vi "Search_Dust_Types.vi"() -> ()   [LabVIEW 2013]
uses:
  Private/Controls/Dust_list.ctl
  <vilib>/Utility/miscctls.llb/LVPointTypeDef.ctl
panel:
  out "Descending":string
  out "Ascending":string
  out "dust_weight text":string
  out "bottle_weight text":string
  out "source_weight text":string
  out "dust_density text":string
  out "dust_name text":string
  out "id_dust_type text":string
  in  "Exit":bool
  out "error out":errorcluster
  in  "error in (no error)":errorcluster
  in  "dust_weight":bool
  in  "bottle_weight":bool
  in  "source_weight":bool
  in  "dust_density":bool
  in  "dust_name":bool
  in  "id_dust_type":bool
  out "Array":T1[](array[typedef])
  # "Size"
  # "Comments"
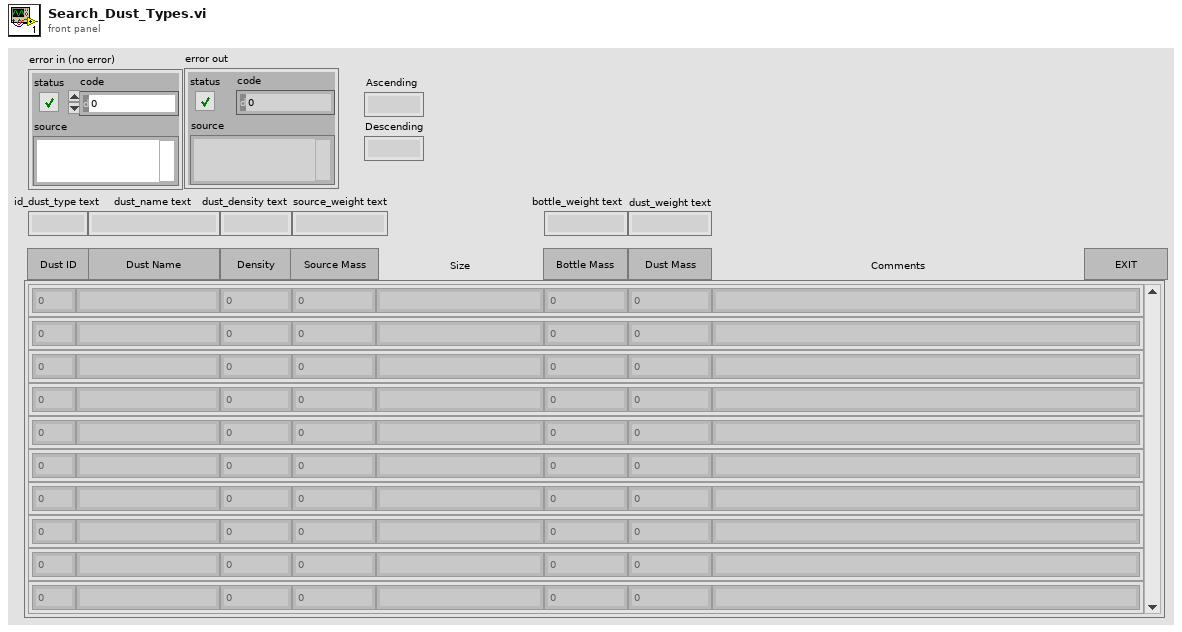
[diagram p1: front panel]
types:
  T1 = typedef "dust_list.ctl" = cluster{"id_dust_type":i32, "dust_name":string, "dust_density":dbl, "source_weight":dbl, "size":string, "bottle_weight":dbl, "dust_mass":dbl, "comments":string}
  T2 = typedef "LVPointTypeDef.ctl" = cluster{"Horizontal":i16, "Vertical":i16}
  T3 = enum16{"dust_name", "dust_density", "source_weight", "bottle_weight", "dust_weight"}
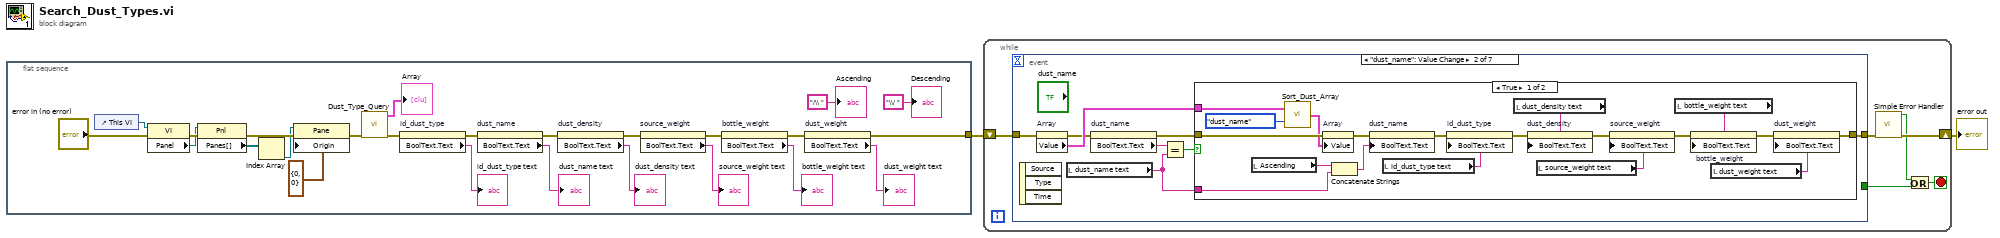
[diagram p0: block diagram]
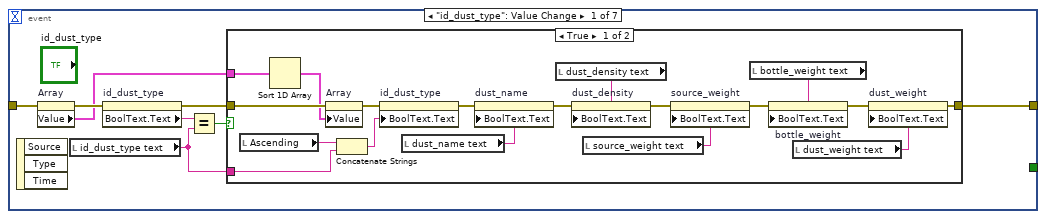
[diagram p2: hidden frame]
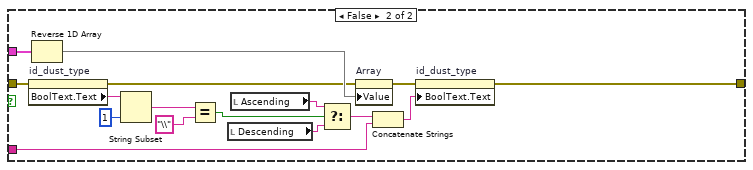
[diagram p3: hidden frame]
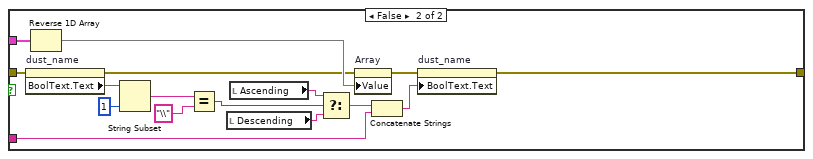
[diagram p4: hidden frame]
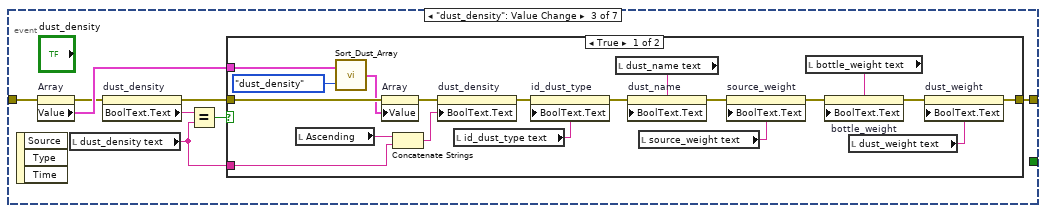
[diagram p5: hidden frame]
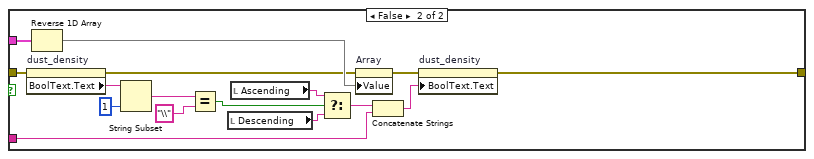
[diagram p6: hidden frame]
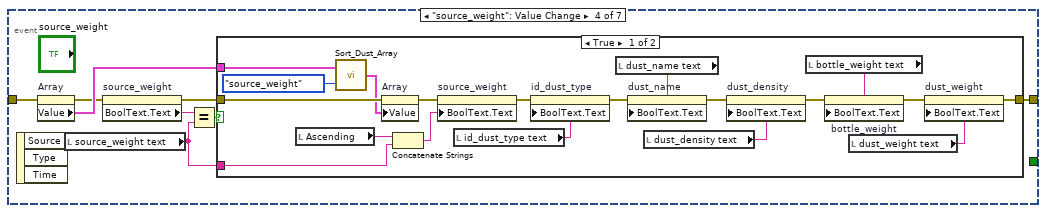
[diagram p7: hidden frame]
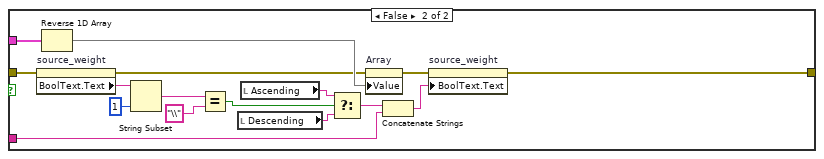
[diagram p8: hidden frame]
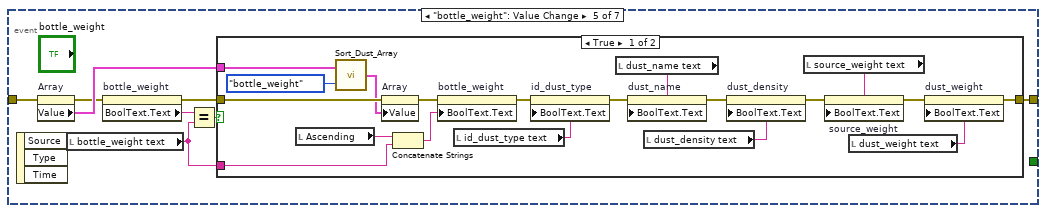
[diagram p9: hidden frame]
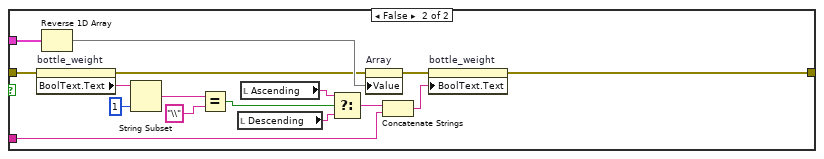
[diagram p10: hidden frame]
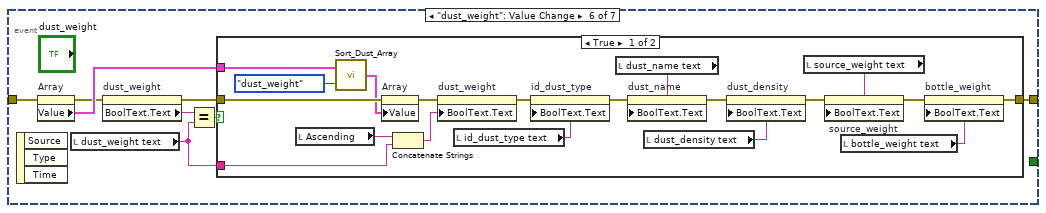
[diagram p11: hidden frame]
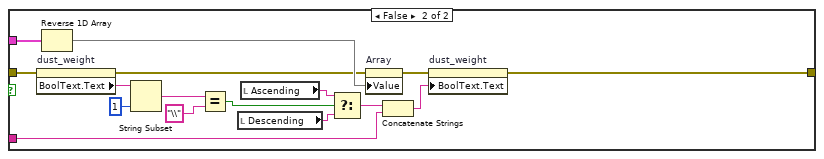
[diagram p12: hidden frame]
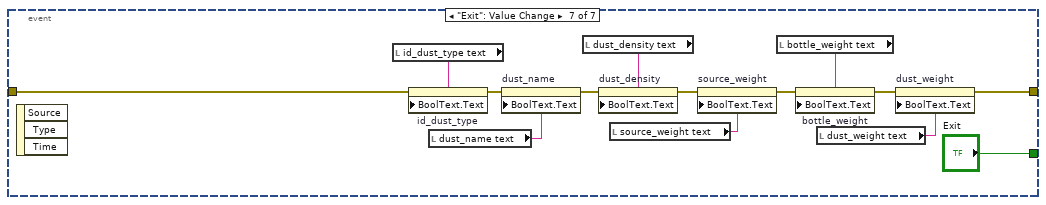
[diagram p13: hidden frame]
diagram:
  n1 = flat-sequence {
    tunnel: [w16] -> w1
    frame #0 {
      n2 = control-ref of="This VI"() -> (w10:refnum<vi>)
      n3 = property class="VI"(reference=w10, error in="error in (no error)") -> (error out=w9:errorcluster, "Panel"=w8:refnum<vi>)  [unwired: 1 out]
      n4 = property class="Pnl"(reference=w8, error in=w9) -> (error out=w7:errorcluster, "Panes[]"=w6:refnum<vi>[])  [unwired: 1 out]
      n5 = Index Array(array=w6) -> (element=w5:refnum<vi>)  [unwired: 1 in]
      n6 = property class="Pane"(reference=w5, error in=w7, "Origin"=T2 {"Horizontal"=0, "Vertical"=0}) -> (error out=w3:errorcluster)  [unwired: 1 out]
      n7 = call "Dust_Type_Query.vi"("error in (no error)"=w3) -> ("error out"=w13:errorcluster, "Dust Type Array"=→"Array":T1[])  [unwired: 9 in]
      n8 = property on="id_dust_type" class="Bool"(error in=w13) -> (error out=w26:errorcluster, "BoolText.Text"=→"id_dust_type text":string)  [unwired: 1 in, 1 out]
      n9 = property on="dust_name" class="Bool"(error in=w26) -> (error out=w25:errorcluster, "BoolText.Text"=→"dust_name text":string)  [unwired: 1 in, 1 out]
      n10 = property on="dust_density" class="Bool"(error in=w25) -> (error out=w22:errorcluster, "BoolText.Text"=→"dust_density text":string)  [unwired: 1 in, 1 out]
      n11 = property on="source_weight" class="Bool"(error in=w22) -> (error out=w20:errorcluster, "BoolText.Text"=→"source_weight text":string)  [unwired: 1 in, 1 out]
      n12 = property on="bottle_weight" class="Bool"(error in=w20) -> (error out=w18:errorcluster, "BoolText.Text"=→"bottle_weight text":string)  [unwired: 1 in, 1 out]
      n13 = property on="dust_weight" class="Bool"(error in=w18) -> (error out=w16:errorcluster, "BoolText.Text"=→"dust_weight text":string)  [unwired: 1 in, 1 out]
      "Ascending" <- "/\\ " ("Ascending")
      "Descending" <- "\\/ " ("Descending")
    }
  }
  n14 = while {
    shift-right: [w30] -> w2
    shift-left: w1 -> [w33]
    stop <- w29 stop-if-true
    n15 = event shown="[1] \"dust_name\": Value Change" {
      selector: _ -> [_ _ _ _ _ _ _]
      dyn-events: _ -> [_ _ _ _ _ _ _]
      timeout: _ -> [_ _ _ _ _ _ _]
      tunnel: w33 -> [w41 w83 w126 w169 w212 w255 w298]
      tunnel: [w40 w82 w125 w168 w211 w254 w297] -> w32
      tunnel: [_ _ _ _ _ _ "Exit"] -> w31
      event "id_dust_type": Value Change {
        n16 = event-data() -> ()  [unwired: 1 in, 3 out]
        n17 = property on="Array" class="Arr (strict)"(error in=w41) -> (error out=w35:errorcluster, "Value"=w34:T1[])  [unwired: 1 in, 1 out]
        n18 = local read "id_dust_type text"() -> (w38:string)
        n19 = property on="id_dust_type" class="Bool"(error in=w35) -> (error out=w36:errorcluster, "BoolText.Text"=w39:string)  [unwired: 1 in, 1 out]
        n20 = Equal?(x=w39, y=w38) -> (x = y?=w37:bool)
        n21 = case shown="True" w37 {
          tunnel: [w46 w74] -> w40
          tunnel: w38 -> [w57 w73]
          tunnel: w36 -> [w45 w62]
          tunnel: w34 -> [w43 w72]
          frame True {
            n22 = local read "Ascending"() -> (w58:string)
            n23 = Sort 1D Array(array=w43) -> (sorted array=w42:T1[])
            n24 = property on="Array" class="Arr (strict)"(error in=w45, "Value"=w42) -> (error out=w44:errorcluster)  [unwired: 1 in, 1 out]
            n25 = Concatenate Strings(w58, w57) -> (w59:string)
            n26 = property on="id_dust_type" class="Bool"(error in=w44, "BoolText.Text"=w59) -> (error out=w47:errorcluster)  [unwired: 1 in, 1 out]
            n27 = local read "dust_name text"() -> (w51:string)
            n28 = property on="dust_name" class="Bool"(error in=w47, "BoolText.Text"=w51) -> (error out=w52:errorcluster)  [unwired: 1 in, 1 out]
            n29 = local read "dust_density text"() -> (w50:string)
            n30 = property on="dust_density" class="Bool"(error in=w52, "BoolText.Text"=w50) -> (error out=w53:errorcluster)  [unwired: 1 in, 1 out]
            n31 = local read "source_weight text"() -> (w49:string)
            n32 = property on="source_weight" class="Bool"(error in=w53, "BoolText.Text"=w49) -> (error out=w54:errorcluster)  [unwired: 1 in, 1 out]
            n33 = local read "bottle_weight text"() -> (w48:string)
            n34 = property on="bottle_weight" class="Bool"(error in=w54, "BoolText.Text"=w48) -> (error out=w55:errorcluster)  [unwired: 1 in, 1 out]
            n35 = local read "dust_weight text"() -> (w56:string)
            n36 = property on="dust_weight" class="Bool"(error in=w55, "BoolText.Text"=w56) -> (error out=w46:errorcluster)  [unwired: 1 in, 1 out]
          }
          frame False {
            n37 = property on="id_dust_type" class="Bool"(error in=w62) -> (error out=w61:errorcluster, "BoolText.Text"=w68:string)  [unwired: 1 in, 1 out]
            n38 = Reverse 1D Array(array=w72) -> (reversed array=w71:T1[])
            n39 = String Subset(string=w68, length (rest)=1 ("length (rest)")) -> (substring=w65:string)  [unwired: 1 in]
            n40 = Equal?(x=w65, y="\\") -> (x = y?=w63:bool)
            n41 = local read "Descending"() -> (w70:string)
            n42 = local read "Ascending"() -> (w66:string)
            n43 = Select(t=w66, s=w63, f=w70) -> (s? t:f=w69:string)
            n44 = property on="Array" class="Arr (strict)"(error in=w61, "Value"=w71) -> (error out=w60:errorcluster)  [unwired: 1 in, 1 out]
            n45 = Concatenate Strings(w69, w73) -> (w75:string)
            n46 = property on="id_dust_type" class="Bool"(error in=w60, "BoolText.Text"=w75) -> (error out=w74:errorcluster)  [unwired: 1 in, 1 out]
          }
        }
      }
      event "dust_name": Value Change {
        n47 = event-data() -> ()  [unwired: 1 in, 3 out]
        n48 = property on="Array" class="Arr (strict)"(error in=w83) -> (error out=w78:errorcluster, "Value"=w79:T1[])  [unwired: 1 in, 1 out]
        n49 = local read "dust_name text"() -> (w81:string)
        n50 = property on="dust_name" class="Bool"(error in=w78) -> (error out=w76:errorcluster, "BoolText.Text"=w77:string)  [unwired: 1 in, 1 out]
        n51 = Equal?(x=w77, y=w81) -> (x = y?=w80:bool)
        n52 = case shown="True" w80 {
          tunnel: [w91 w104] -> w82
          tunnel: w81 -> [w101 w118]
          tunnel: w76 -> [w90 w108]
          tunnel: w79 -> [w89 w117]
          frame True {
            n53 = local read "Ascending"() -> (w102:string)
            n54 = call "Sort_Dust_Array.vi"("Order by..."=T3."dust_name", "Array In"=w89) -> ("Array out"=w88:T1[])
            n55 = property on="Array" class="Arr (strict)"(error in=w90, "Value"=w88) -> (error out=w86:errorcluster)  [unwired: 1 in, 1 out]
            n56 = Concatenate Strings(w102, w101) -> (w85:string)
            n57 = property on="dust_name" class="Bool"(error in=w86, "BoolText.Text"=w85) -> (error out=w87:errorcluster)  [unwired: 1 in, 1 out]
            n58 = local read "id_dust_type text"() -> (w95:string)
            n59 = property on="id_dust_type" class="Bool"(error in=w87, "BoolText.Text"=w95) -> (error out=w96:errorcluster)  [unwired: 1 in, 1 out]
            n60 = local read "dust_density text"() -> (w94:string)
            n61 = property on="dust_density" class="Bool"(error in=w96, "BoolText.Text"=w94) -> (error out=w97:errorcluster)  [unwired: 1 in, 1 out]
            n62 = local read "source_weight text"() -> (w93:string)
            n63 = property on="source_weight" class="Bool"(error in=w97, "BoolText.Text"=w93) -> (error out=w98:errorcluster)  [unwired: 1 in, 1 out]
            n64 = local read "bottle_weight text"() -> (w92:string)
            n65 = property on="bottle_weight" class="Bool"(error in=w98, "BoolText.Text"=w92) -> (error out=w99:errorcluster)  [unwired: 1 in, 1 out]
            n66 = local read "dust_weight text"() -> (w100:string)
            n67 = property on="dust_weight" class="Bool"(error in=w99, "BoolText.Text"=w100) -> (error out=w91:errorcluster)  [unwired: 1 in, 1 out]
          }
          frame False {
            n68 = property on="dust_name" class="Bool"(error in=w108) -> (error out=w107:errorcluster, "BoolText.Text"=w106:string)  [unwired: 1 in, 1 out]
            n69 = Reverse 1D Array(array=w117) -> (reversed array=w116:T1[])
            n70 = String Subset(string=w106, length (rest)=1 ("length (rest)")) -> (substring=w111:string)  [unwired: 1 in]
            n71 = Equal?(x=w111, y="\\") -> (x = y?=w109:bool)
            n72 = local read "Descending"() -> (w115:string)
            n73 = local read "Ascending"() -> (w112:string)
            n74 = Select(t=w112, s=w109, f=w115) -> (s? t:f=w114:string)
            n75 = property on="Array" class="Arr (strict)"(error in=w107, "Value"=w116) -> (error out=w105:errorcluster)  [unwired: 1 in, 1 out]
            n76 = Concatenate Strings(w114, w118) -> (w103:string)
            n77 = property on="dust_name" class="Bool"(error in=w105, "BoolText.Text"=w103) -> (error out=w104:errorcluster)  [unwired: 1 in, 1 out]
          }
        }
      }
      event "dust_density": Value Change {
        n78 = event-data() -> ()  [unwired: 1 in, 3 out]
        n79 = property on="Array" class="Arr (strict)"(error in=w126) -> (error out=w121:errorcluster, "Value"=w122:T1[])  [unwired: 1 in, 1 out]
        n80 = local read "dust_density text"() -> (w124:string)
        n81 = property on="dust_density" class="Bool"(error in=w121) -> (error out=w119:errorcluster, "BoolText.Text"=w120:string)  [unwired: 1 in, 1 out]
        n82 = Equal?(x=w120, y=w124) -> (x = y?=w123:bool)
        n83 = case shown="True" w123 {
          tunnel: [w134 w147] -> w125
          tunnel: w124 -> [w144 w161]
          tunnel: w119 -> [w133 w151]
          tunnel: w122 -> [w132 w160]
          frame True {
            n84 = local read "Ascending"() -> (w145:string)
            n85 = call "Sort_Dust_Array.vi"("Order by..."=T3."dust_density", "Array In"=w132) -> ("Array out"=w131:T1[])
            n86 = property on="Array" class="Arr (strict)"(error in=w133, "Value"=w131) -> (error out=w129:errorcluster)  [unwired: 1 in, 1 out]
            n87 = Concatenate Strings(w145, w144) -> (w128:string)
            n88 = property on="dust_density" class="Bool"(error in=w129, "BoolText.Text"=w128) -> (error out=w130:errorcluster)  [unwired: 1 in, 1 out]
            n89 = local read "id_dust_type text"() -> (w138:string)
            n90 = property on="id_dust_type" class="Bool"(error in=w130, "BoolText.Text"=w138) -> (error out=w139:errorcluster)  [unwired: 1 in, 1 out]
            n91 = local read "dust_name text"() -> (w137:string)
            n92 = property on="dust_name" class="Bool"(error in=w139, "BoolText.Text"=w137) -> (error out=w140:errorcluster)  [unwired: 1 in, 1 out]
            n93 = local read "source_weight text"() -> (w136:string)
            n94 = property on="source_weight" class="Bool"(error in=w140, "BoolText.Text"=w136) -> (error out=w141:errorcluster)  [unwired: 1 in, 1 out]
            n95 = local read "bottle_weight text"() -> (w135:string)
            n96 = property on="bottle_weight" class="Bool"(error in=w141, "BoolText.Text"=w135) -> (error out=w142:errorcluster)  [unwired: 1 in, 1 out]
            n97 = local read "dust_weight text"() -> (w143:string)
            n98 = property on="dust_weight" class="Bool"(error in=w142, "BoolText.Text"=w143) -> (error out=w134:errorcluster)  [unwired: 1 in, 1 out]
          }
          frame False {
            n99 = property on="dust_density" class="Bool"(error in=w151) -> (error out=w150:errorcluster, "BoolText.Text"=w149:string)  [unwired: 1 in, 1 out]
            n100 = Reverse 1D Array(array=w160) -> (reversed array=w159:T1[])
            n101 = String Subset(string=w149, length (rest)=1 ("length (rest)")) -> (substring=w154:string)  [unwired: 1 in]
            n102 = Equal?(x=w154, y="\\") -> (x = y?=w152:bool)
            n103 = local read "Descending"() -> (w158:string)
            n104 = local read "Ascending"() -> (w155:string)
            n105 = Select(t=w155, s=w152, f=w158) -> (s? t:f=w157:string)
            n106 = property on="Array" class="Arr (strict)"(error in=w150, "Value"=w159) -> (error out=w148:errorcluster)  [unwired: 1 in, 1 out]
            n107 = Concatenate Strings(w157, w161) -> (w146:string)
            n108 = property on="dust_density" class="Bool"(error in=w148, "BoolText.Text"=w146) -> (error out=w147:errorcluster)  [unwired: 1 in, 1 out]
          }
        }
      }
      event "source_weight": Value Change {
        n109 = event-data() -> ()  [unwired: 1 in, 3 out]
        n110 = property on="Array" class="Arr (strict)"(error in=w169) -> (error out=w164:errorcluster, "Value"=w165:T1[])  [unwired: 1 in, 1 out]
        n111 = local read "source_weight text"() -> (w167:string)
        n112 = property on="source_weight" class="Bool"(error in=w164) -> (error out=w162:errorcluster, "BoolText.Text"=w163:string)  [unwired: 1 in, 1 out]
        n113 = Equal?(x=w163, y=w167) -> (x = y?=w166:bool)
        n114 = case shown="True" w166 {
          tunnel: [w177 w190] -> w168
          tunnel: w167 -> [w187 w204]
          tunnel: w162 -> [w176 w194]
          tunnel: w165 -> [w175 w203]
          frame True {
            n115 = local read "Ascending"() -> (w188:string)
            n116 = call "Sort_Dust_Array.vi"("Order by..."=T3."source_weight", "Array In"=w175) -> ("Array out"=w174:T1[])
            n117 = property on="Array" class="Arr (strict)"(error in=w176, "Value"=w174) -> (error out=w172:errorcluster)  [unwired: 1 in, 1 out]
            n118 = Concatenate Strings(w188, w187) -> (w171:string)
            n119 = property on="source_weight" class="Bool"(error in=w172, "BoolText.Text"=w171) -> (error out=w173:errorcluster)  [unwired: 1 in, 1 out]
            n120 = local read "id_dust_type text"() -> (w181:string)
            n121 = property on="id_dust_type" class="Bool"(error in=w173, "BoolText.Text"=w181) -> (error out=w182:errorcluster)  [unwired: 1 in, 1 out]
            n122 = local read "dust_name text"() -> (w180:string)
            n123 = property on="dust_name" class="Bool"(error in=w182, "BoolText.Text"=w180) -> (error out=w183:errorcluster)  [unwired: 1 in, 1 out]
            n124 = local read "dust_density text"() -> (w179:string)
            n125 = property on="dust_density" class="Bool"(error in=w183, "BoolText.Text"=w179) -> (error out=w184:errorcluster)  [unwired: 1 in, 1 out]
            n126 = local read "bottle_weight text"() -> (w178:string)
            n127 = property on="bottle_weight" class="Bool"(error in=w184, "BoolText.Text"=w178) -> (error out=w185:errorcluster)  [unwired: 1 in, 1 out]
            n128 = local read "dust_weight text"() -> (w186:string)
            n129 = property on="dust_weight" class="Bool"(error in=w185, "BoolText.Text"=w186) -> (error out=w177:errorcluster)  [unwired: 1 in, 1 out]
          }
          frame False {
            n130 = property on="source_weight" class="Bool"(error in=w194) -> (error out=w193:errorcluster, "BoolText.Text"=w192:string)  [unwired: 1 in, 1 out]
            n131 = Reverse 1D Array(array=w203) -> (reversed array=w202:T1[])
            n132 = String Subset(string=w192, length (rest)=1 ("length (rest)")) -> (substring=w197:string)  [unwired: 1 in]
            n133 = Equal?(x=w197, y="\\") -> (x = y?=w195:bool)
            n134 = local read "Descending"() -> (w201:string)
            n135 = local read "Ascending"() -> (w198:string)
            n136 = Select(t=w198, s=w195, f=w201) -> (s? t:f=w200:string)
            n137 = property on="Array" class="Arr (strict)"(error in=w193, "Value"=w202) -> (error out=w191:errorcluster)  [unwired: 1 in, 1 out]
            n138 = Concatenate Strings(w200, w204) -> (w189:string)
            n139 = property on="source_weight" class="Bool"(error in=w191, "BoolText.Text"=w189) -> (error out=w190:errorcluster)  [unwired: 1 in, 1 out]
          }
        }
      }
      event "bottle_weight": Value Change {
        n140 = event-data() -> ()  [unwired: 1 in, 3 out]
        n141 = property on="Array" class="Arr (strict)"(error in=w212) -> (error out=w207:errorcluster, "Value"=w208:T1[])  [unwired: 1 in, 1 out]
        n142 = local read "bottle_weight text"() -> (w210:string)
        n143 = property on="bottle_weight" class="Bool"(error in=w207) -> (error out=w205:errorcluster, "BoolText.Text"=w206:string)  [unwired: 1 in, 1 out]
        n144 = Equal?(x=w206, y=w210) -> (x = y?=w209:bool)
        n145 = case shown="True" w209 {
          tunnel: [w220 w233] -> w211
          tunnel: w210 -> [w230 w247]
          tunnel: w205 -> [w219 w237]
          tunnel: w208 -> [w218 w246]
          frame True {
            n146 = local read "Ascending"() -> (w231:string)
            n147 = call "Sort_Dust_Array.vi"("Order by..."=T3."bottle_weight", "Array In"=w218) -> ("Array out"=w217:T1[])
            n148 = property on="Array" class="Arr (strict)"(error in=w219, "Value"=w217) -> (error out=w215:errorcluster)  [unwired: 1 in, 1 out]
            n149 = Concatenate Strings(w231, w230) -> (w214:string)
            n150 = property on="bottle_weight" class="Bool"(error in=w215, "BoolText.Text"=w214) -> (error out=w216:errorcluster)  [unwired: 1 in, 1 out]
            n151 = local read "id_dust_type text"() -> (w224:string)
            n152 = property on="id_dust_type" class="Bool"(error in=w216, "BoolText.Text"=w224) -> (error out=w225:errorcluster)  [unwired: 1 in, 1 out]
            n153 = local read "dust_name text"() -> (w223:string)
            n154 = property on="dust_name" class="Bool"(error in=w225, "BoolText.Text"=w223) -> (error out=w226:errorcluster)  [unwired: 1 in, 1 out]
            n155 = local read "dust_density text"() -> (w222:string)
            n156 = property on="dust_density" class="Bool"(error in=w226, "BoolText.Text"=w222) -> (error out=w227:errorcluster)  [unwired: 1 in, 1 out]
            n157 = local read "source_weight text"() -> (w221:string)
            n158 = property on="source_weight" class="Bool"(error in=w227, "BoolText.Text"=w221) -> (error out=w228:errorcluster)  [unwired: 1 in, 1 out]
            n159 = local read "dust_weight text"() -> (w229:string)
            n160 = property on="dust_weight" class="Bool"(error in=w228, "BoolText.Text"=w229) -> (error out=w220:errorcluster)  [unwired: 1 in, 1 out]
          }
          frame False {
            n161 = property on="bottle_weight" class="Bool"(error in=w237) -> (error out=w236:errorcluster, "BoolText.Text"=w235:string)  [unwired: 1 in, 1 out]
            n162 = Reverse 1D Array(array=w246) -> (reversed array=w245:T1[])
            n163 = String Subset(string=w235, length (rest)=1 ("length (rest)")) -> (substring=w240:string)  [unwired: 1 in]
            n164 = Equal?(x=w240, y="\\") -> (x = y?=w238:bool)
            n165 = local read "Descending"() -> (w244:string)
            n166 = local read "Ascending"() -> (w241:string)
            n167 = Select(t=w241, s=w238, f=w244) -> (s? t:f=w243:string)
            n168 = property on="Array" class="Arr (strict)"(error in=w236, "Value"=w245) -> (error out=w234:errorcluster)  [unwired: 1 in, 1 out]
            n169 = Concatenate Strings(w243, w247) -> (w232:string)
            n170 = property on="bottle_weight" class="Bool"(error in=w234, "BoolText.Text"=w232) -> (error out=w233:errorcluster)  [unwired: 1 in, 1 out]
          }
        }
      }
      event "dust_weight": Value Change {
        n171 = event-data() -> ()  [unwired: 1 in, 3 out]
        n172 = property on="Array" class="Arr (strict)"(error in=w255) -> (error out=w250:errorcluster, "Value"=w251:T1[])  [unwired: 1 in, 1 out]
        n173 = local read "dust_weight text"() -> (w253:string)
        n174 = property on="dust_weight" class="Bool"(error in=w250) -> (error out=w248:errorcluster, "BoolText.Text"=w249:string)  [unwired: 1 in, 1 out]
        n175 = Equal?(x=w249, y=w253) -> (x = y?=w252:bool)
        n176 = case shown="True" w252 {
          tunnel: [w263 w276] -> w254
          tunnel: w253 -> [w273 w290]
          tunnel: w248 -> [w262 w280]
          tunnel: w251 -> [w261 w289]
          frame True {
            n177 = local read "Ascending"() -> (w274:string)
            n178 = call "Sort_Dust_Array.vi"("Order by..."=T3."dust_weight", "Array In"=w261) -> ("Array out"=w260:T1[])
            n179 = property on="Array" class="Arr (strict)"(error in=w262, "Value"=w260) -> (error out=w258:errorcluster)  [unwired: 1 in, 1 out]
            n180 = Concatenate Strings(w274, w273) -> (w257:string)
            n181 = property on="dust_weight" class="Bool"(error in=w258, "BoolText.Text"=w257) -> (error out=w259:errorcluster)  [unwired: 1 in, 1 out]
            n182 = local read "id_dust_type text"() -> (w267:string)
            n183 = property on="id_dust_type" class="Bool"(error in=w259, "BoolText.Text"=w267) -> (error out=w268:errorcluster)  [unwired: 1 in, 1 out]
            n184 = local read "dust_name text"() -> (w266:string)
            n185 = property on="dust_name" class="Bool"(error in=w268, "BoolText.Text"=w266) -> (error out=w269:errorcluster)  [unwired: 1 in, 1 out]
            n186 = local read "dust_density text"() -> (w265:string)
            n187 = property on="dust_density" class="Bool"(error in=w269, "BoolText.Text"=w265) -> (error out=w270:errorcluster)  [unwired: 1 in, 1 out]
            n188 = local read "source_weight text"() -> (w264:string)
            n189 = property on="source_weight" class="Bool"(error in=w270, "BoolText.Text"=w264) -> (error out=w271:errorcluster)  [unwired: 1 in, 1 out]
            n190 = local read "bottle_weight text"() -> (w272:string)
            n191 = property on="bottle_weight" class="Bool"(error in=w271, "BoolText.Text"=w272) -> (error out=w263:errorcluster)  [unwired: 1 in, 1 out]
          }
          frame False {
            n192 = property on="dust_weight" class="Bool"(error in=w280) -> (error out=w279:errorcluster, "BoolText.Text"=w278:string)  [unwired: 1 in, 1 out]
            n193 = Reverse 1D Array(array=w289) -> (reversed array=w288:T1[])
            n194 = String Subset(string=w278, length (rest)=1 ("length (rest)")) -> (substring=w283:string)  [unwired: 1 in]
            n195 = Equal?(x=w283, y="\\") -> (x = y?=w281:bool)
            n196 = local read "Descending"() -> (w287:string)
            n197 = local read "Ascending"() -> (w284:string)
            n198 = Select(t=w284, s=w281, f=w287) -> (s? t:f=w286:string)
            n199 = property on="Array" class="Arr (strict)"(error in=w279, "Value"=w288) -> (error out=w277:errorcluster)  [unwired: 1 in, 1 out]
            n200 = Concatenate Strings(w286, w290) -> (w275:string)
            n201 = property on="dust_weight" class="Bool"(error in=w277, "BoolText.Text"=w275) -> (error out=w276:errorcluster)  [unwired: 1 in, 1 out]
          }
        }
      }
      event "Exit": Value Change {
        n202 = event-data() -> ()  [unwired: 1 in, 3 out]
        n203 = local read "id_dust_type text"() -> (w296:string)
        n204 = property on="id_dust_type" class="Bool"(error in=w298, "BoolText.Text"=w296) -> (error out=w299:errorcluster)  [unwired: 1 in, 1 out]
        n205 = local read "dust_name text"() -> (w295:string)
        n206 = property on="dust_name" class="Bool"(error in=w299, "BoolText.Text"=w295) -> (error out=w300:errorcluster)  [unwired: 1 in, 1 out]
        n207 = local read "dust_density text"() -> (w294:string)
        n208 = property on="dust_density" class="Bool"(error in=w300, "BoolText.Text"=w294) -> (error out=w301:errorcluster)  [unwired: 1 in, 1 out]
        n209 = local read "source_weight text"() -> (w293:string)
        n210 = property on="source_weight" class="Bool"(error in=w301, "BoolText.Text"=w293) -> (error out=w302:errorcluster)  [unwired: 1 in, 1 out]
        n211 = local read "bottle_weight text"() -> (w292:string)
        n212 = property on="bottle_weight" class="Bool"(error in=w302, "BoolText.Text"=w292) -> (error out=w303:errorcluster)  [unwired: 1 in, 1 out]
        n213 = local read "dust_weight text"() -> (w291:string)
        n214 = property on="dust_weight" class="Bool"(error in=w303, "BoolText.Text"=w291) -> (error out=w297:errorcluster)  [unwired: 1 in, 1 out]
      }
    }
    n215 = call <vilib>:"Simple Error Handler.vi"("error in (no error)"=w32) -> ("error?"=w28:bool, "error out"=w30:errorcluster)  [unwired: 4 in, 3 out]
    n216 = Or(x=w28, y=w31) -> (x .or. y?=w29:bool)
  }
  "error out" <- w2
